vi "Pressure Cal Point.vi"(8 "Condition":string[][](array[string]), 9 "인덱스 (열)":i32, 11 "교정방법":string) -> (0 "배열":string[][](array[string]), 1 "단위":string, 2 "최소용량":string, 3 "최대용량":string)   [LabVIEW 2020]
uses:
  Variables/Global_Cal Info.vi
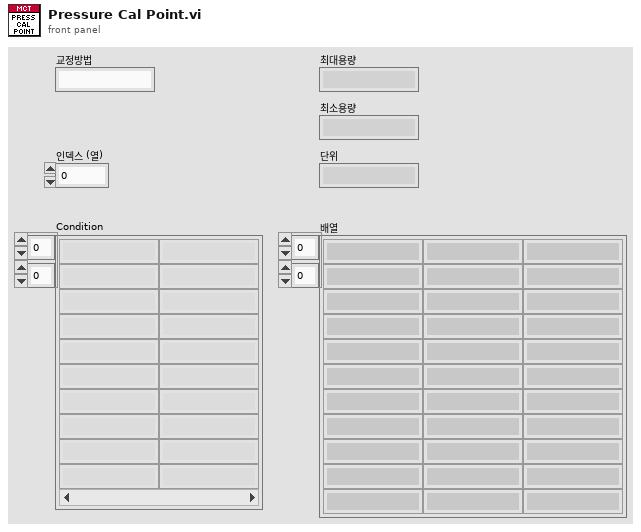
[diagram p1: front panel]
types:
  T1 = cluster{"세부분류코드":string, "형식":string, "옵션":string, "측정기명":string, "EXCEL파일명":string, "TEMP":string}
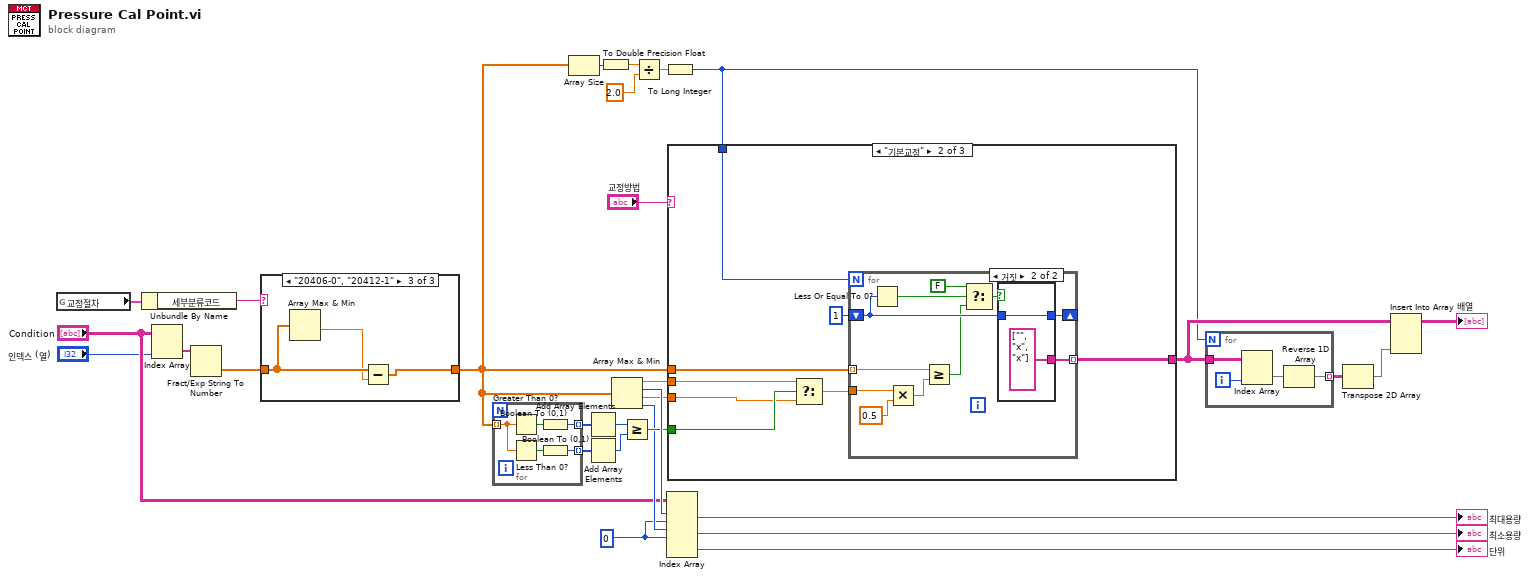
[diagram p0: block diagram]
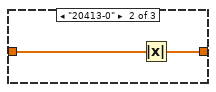
[diagram p3: hidden frame]
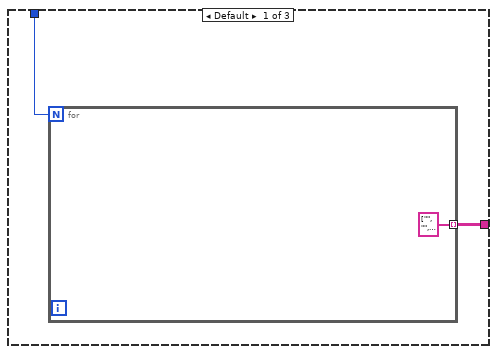
[diagram p4: hidden frame]
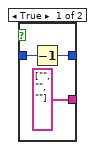
[diagram p5: hidden frame]
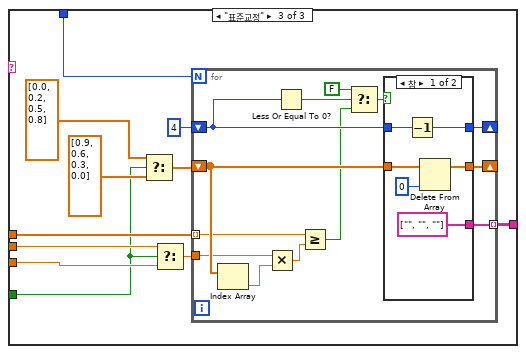
[diagram p6: hidden frame]
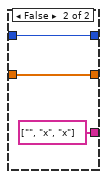
[diagram p7: hidden frame]
diagram:
  w5 = 0 ("인덱스 (열)")
  n1 = global read "Global_Cal Info.vi" "교정절차"() -> (w2:T1)
  n2 = Unbundle By Name(w2) -> ("세부분류코드"=w1:string)
  n3 = Index Array(array="Condition", index (col)="인덱스 (열)") -> (element=w25:string[])  [unwired: 1 in]
  n4 = Fract/Exp String To Number(string=w25) -> (number=w4:dbl[])  [unwired: 3 in, 1 out]
  n5 = case shown="\"20406-0\", \"20412-1\"" w1 {
    tunnel: w4 -> [w31 w33 w36]
    tunnel: [w31 w32 w34] -> w3
    frame Default {
    }
    frame "20413-0" {
      n6 = Absolute Value(x=w33) -> (abs(x)=w32:dbl[])
    }
    frame "20406-0", "20412-1" {
      n7 = Array Max & Min(array=w36) -> (min value=w35:dbl)  [unwired: 3 out]
      n8 = Subtract(x=w36, y=w35) -> (x-y=w34:dbl[])
    }
  }
  n9 = for {
    tunnel: w3 -> [w41] mode=indexing
    tunnel: [w38] -> w13 mode=indexing
    tunnel: [w37] -> w14 mode=indexing
    n10 = Greater Than 0?(x=w41) -> (x > 0?=w40:bool)
    n11 = Less Than 0?(x=w41) -> (x < 0?=w39:bool)
    n12 = Boolean To (0,1)(Boolean=w40) -> (0, 1=w38:i16)
    n13 = Boolean To (0,1)(Boolean=w39) -> (0, 1=w37:i16)
  }
  n14 = Array Size(array=w3) -> (size(s)=w30:i32)
  n15 = Add Array Elements(numeric array=w13) -> (sum=w15:i16)
  n16 = Add Array Elements(numeric array=w14) -> (sum=w16:i16)
  n17 = To Double Precision Float(number=w30) -> (double precision float=w28:dbl)
  n18 = Array Max & Min(array=w3) -> (max value=w29:dbl, max index (indices)=w18:i32, min value=w11:dbl, min index (indices)=w9:i32)
  n19 = Greater Or Equal?(x=w15, y=w16) -> (x >= y?=w12:bool)
  n20 = Divide(x=w28, y=2.0) -> (x/y=w27:dbl)
  n21 = To Long Integer(number=w27) -> (32bit integer=w20:i32)
  n22 = Index Array(array="Condition", index (row) #1=w18, index (col) #1=w5, index (row) #2=w9, index (col) #2=w5) -> (element #1=→"최대용량":string, element #2=→"최소용량":string, element #3=→"단위":string)  [unwired: 2 in]
  n23 = case shown="\"기본교정\"" "교정방법" {
    tunnel: w3 -> [_ w48 w79]
    tunnel: w29 -> [_ w47 w74]
    tunnel: w20 -> [w42 w49 w77]
    tunnel: [w43 w50 w76] -> w21
    tunnel: w12 -> [_ w46 w69]
    tunnel: w11 -> [_ w45 w73]
    frame Default {
      n24 = for {
        N: w42 -> [_]
        tunnel: [string[] ["", "", ""]] -> w43 mode=indexing
      }
    }
    frame "기본교정" {
      n25 = Select(t=w47, s=w46, f=w45) -> (s? t:f=w52:dbl)
      n26 = for {
        N: w49 -> [_]
        tunnel: w48 -> [w55] mode=indexing
        tunnel: w52 -> [w62]
        shift-right: [w60] -> _
        shift-left: 1 -> [w59]
        tunnel: [w63] -> w50 mode=indexing
        n27 = Less Or Equal To 0?(x=w59) -> (x <= 0?=w58:bool)
        n28 = Multiply(x=w62, y=0.5) -> (x*y=w54:dbl)
        n29 = Greater Or Equal?(x=w55, y=w54) -> (x >= y?=w53:bool)
        n30 = Select(t=FALSE, s=w58, f=w53) -> (s? t:f=w57:bool)
        n31 = case shown="거짓" w57 {
          tunnel: [string[] ["", "", ""] string[] ["", "ⅹ", "ⅹ"]] -> w63
          tunnel: w59 -> [w65 w68]
          tunnel: [w64 w68] -> w60
          frame True {
            n32 = Decrement(x=w65) -> (x-1=w64:i32)
          }
          frame False {
          }
        }
      }
    }
    frame "표준교정" {
      n33 = Select(t=dbl[] [0.0, 0.2, 0.5, 0.8], s=w69, f=dbl[] [0.9, 0.6, 0.3, 0.0]) -> (s? t:f=w70:dbl[])
      n34 = Select(t=w74, s=w69, f=w73) -> (s? t:f=w75:dbl)
      n35 = for {
        N: w77 -> [_]
        tunnel: w79 -> [w82] mode=indexing
        tunnel: w75 -> [w81]
        shift-right: [w91] -> _
        shift-left: 4 -> [w90]
        tunnel: [w92] -> w76 mode=indexing
        shift-right: [w84] -> _
        shift-left: w70 -> [w85]
        n36 = Index Array(array=w85) -> (element=w86:dbl)  [unwired: 1 in]
        n37 = Multiply(x=w81, y=w86) -> (x*y=w80:dbl)
        n38 = Less Or Equal To 0?(x=w90) -> (x <= 0?=w89:bool)
        n39 = Greater Or Equal?(x=w82, y=w80) -> (x >= y?=w83:bool)
        n40 = Select(t=FALSE, s=w89, f=w83) -> (s? t:f=w88:bool)
        n41 = case shown="참" w88 {
          tunnel: [string[] ["", "", ""] string[] ["", "ⅹ", "ⅹ"]] -> w92
          tunnel: w90 -> [w97 w100]
          tunnel: [w96 w100] -> w91
          tunnel: w85 -> [w95 w99]
          tunnel: [w94 w99] -> w84
          frame True {
            n42 = Decrement(x=w97) -> (x-1=w96:i32)
            n43 = Delete From Array(array=w95, index=0 ("인덱스")) -> (array with subset deleted=w94:dbl[])  [unwired: 1 in, 1 out]
          }
          frame False {
          }
        }
      }
    }
  }
  n44 = for {
    N: w20 -> [_]
    tunnel: w21 -> [w105]
    tunnel: [w102] -> w19 mode=indexing
    i -> [w104]
    n45 = Index Array(array=w105, index (col)=w104) -> (element=w103:string[])  [unwired: 1 in]
    n46 = Reverse 1D Array(array=w103) -> (reversed array=w102:string[])
  }
  n47 = Transpose 2D Array(2D array=w19) -> (transposed array=w22:string[][])
  n48 = Insert Into Array(array=w21, new element=w22) -> (→"배열":string[][])  [unwired: 2 in]
